vi "DAC Run.vi"(8 "error in":errorcluster, 11 "DAC HeatFlow AIV in":refnum<class "DAC HeatFlow AIV.lvclass">) -> (0 "error out":errorcluster, 3 "DAC HeatFlow AIV out":refnum<class "DAC HeatFlow AIV.lvclass">)   [LabVIEW 2019, in "DAC.lvlib" / "DAC HeatFlow AIV.lvclass"]
uses:
  DAC HeatFlow AIV.lvclass
  C:/Users/wg/Documents/LV_Projects/test-stand/App/DAC/DAC.lvclass
  DAC.lvclass/DAC.ctl
  DAC HeatFlow AIV.lvclass/DAC HeatFlow AIV.ctl
  <vilib>/DAQmx/read.llb/DAQmx Read (Analog Wfm 1Chan NSamp).vi
  <vilib>/Analysis/baseanly.llb/Mean (DBL).vi
  <vilib>/DAQmx/miscellaneous.llb/DAQmx Fill In Error Info.vi
  DAC.lvclass
  <vilib>/Analysis/NI_AALBase.lvlib
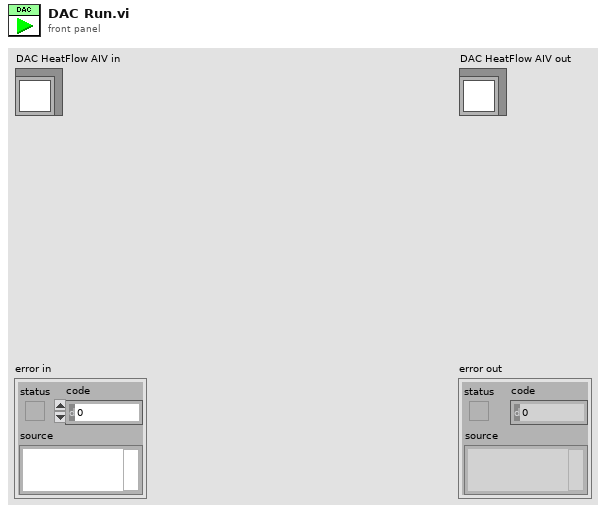
[diagram p1: front panel]
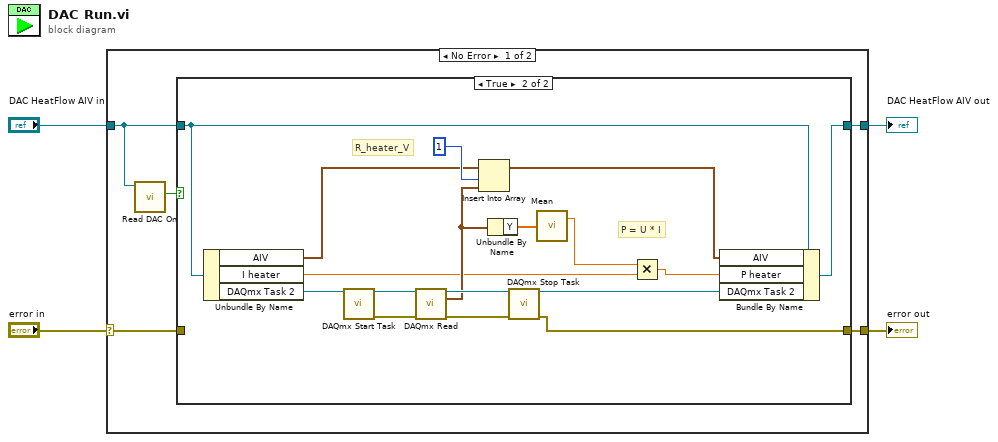
[diagram p0: block diagram]
diagram:
  n1 = case shown="No Error" "error in" {
    selector: "error in" -> [w7 w30]
    tunnel: [w6 w30] -> w2
    tunnel: [w8 w29] -> w1
    tunnel: "DAC HeatFlow AIV in" -> [w5 w29]
    frame No Error {
      n2 = call "Read DAC On.vi"("DAC in"=w5) -> ("DAC On"=w9:bool)  [unwired: 8 in, 2 out]
      n3 = case shown="True" w9 {
        tunnel: w5 -> [w11 w21]
        tunnel: [w11 w23] -> w8
        tunnel: w7 -> [w10 _]
        tunnel: [w10 w14] -> w6
        frame False {
        }
        frame True {
          # "P = U * I"
          # "R_heater_V"
          n4 = Unbundle By Name(w21) -> ("AIV"=w13:waveform(dbl)[], "I heater"=w12:dbl, "DAQmx Task 2"=w28:refnum<k21>)
          n5 = call <vilib>:"DAQmx Start Task.vi"("task/channels in"=w28) -> ("task out"=w27:refnum<k21>, "error out"=w25:errorcluster)  [unwired: 13 in]
          n6 = call-poly <vilib>:"DAQmx Read.vi"("task/channels in"=w27, "error in"=w25) -> ("task out"=w26:refnum<k21>, "data"=w18:waveform(dbl), "error out"=w24:errorcluster)  [unwired: 11 in]
          n7 = Insert Into Array "Insert Into Array"(array=w13, index=1, new element=w18) -> (w15:waveform(dbl)[])
          n8 = Unbundle By Name(w18) -> ("Y"=w19:dbl[])
          n9 = call <vilib>:"DAQmx Stop Task.vi"("task/channels in"=w26, "error in"=w24) -> ("task out"=w22:refnum<k21>, "error out"=w14:errorcluster)  [unwired: 12 in]
          n10 = call-poly <vilib>:"Mean.vi"("X"=w19) -> ("mean"=w17:dbl)  [unwired: 1 out]
          n11 = Multiply(x=w17, y=w12) -> (x*y=w16:dbl)
          n12 = Bundle By Name(cluster=w21, "AIV"=w15, "P heater"=w16, "DAQmx Task 2"=w22) -> (w23:refnum<class "DAC HeatFlow AIV.lvclass">)
        }
      }
    }
    frame Error {
    }
  }
  "error out" <- w2
  "DAC HeatFlow AIV out" <- w1
